vi "Read Element.vi"(8 "error in (no error)":errorcluster, 11 "Vector_DBL in":refnum<class "Vector_DBL.lvclass">) -> (0 "error out":errorcluster, 2 "Element":dbl, 3 "Vector_DBL out":refnum<class "Vector_DBL.lvclass">)   [LabVIEW 2021, in "Vector_DBL.lvclass"]
uses:
  Vector_DBL.lvclass
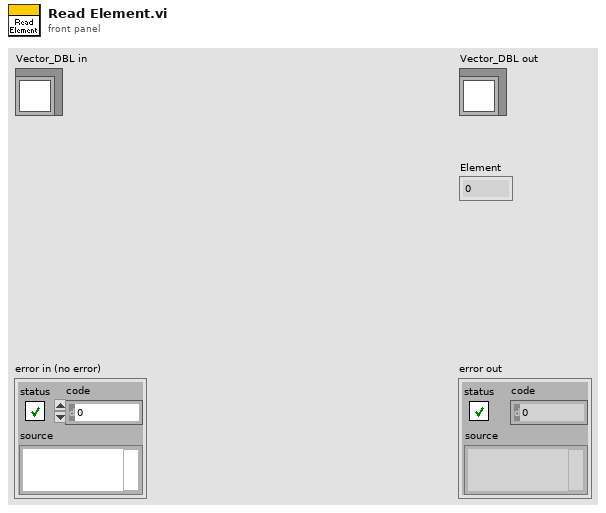
[diagram p1: front panel]
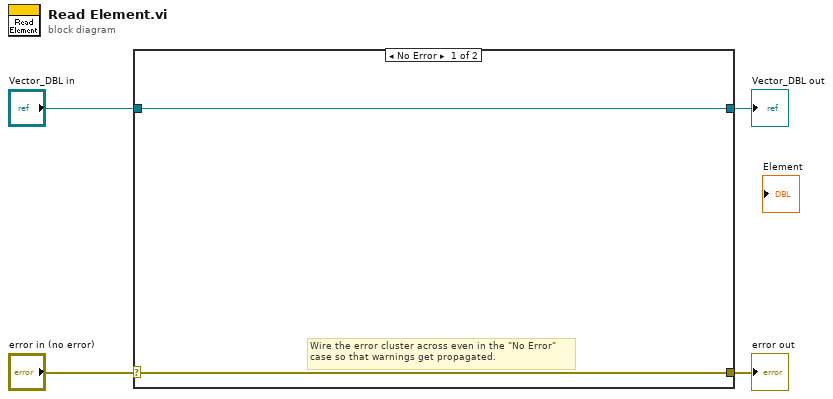
[diagram p0: block diagram]
diagram:
  n1 = case shown="No Error" "error in (no error)" {
    selector: "error in (no error)" -> [w5 w8]
    tunnel: [w5 w8] -> w3
    tunnel: [w6 w7] -> w1
    tunnel: "Vector_DBL in" -> [w6 w7]
    frame No Error {
      # "Wire the error cluster across even in the \"No Error\"\ncase so that warnings get propagated."
    }
    frame Error {
    }
  }
  "error out" <- w3
  "Vector_DBL out" <- w1
